vi "video.add.request.vi"(8 "error in":errorcluster, 9 "Series Tags":map{string, string}(c390), 10 "Video RID":string, 11 "DataScope Name":string="default") -> (0 "error out":errorcluster, 3 "Request":string)   [LabVIEW 2020, in "asset.lvclass"]
uses:
  d09293c4-a5fb-4d14-8e4d-efc786611564.vi
  dbf372a7-e192-454a-a0bf-8f356cd897b9.vi
  <vilib>/JDP Science/JSONtext/Variant to JSON Text.vi
  <vilib>/JDP Science/JSONtext/LVClass Serializer/JSONtext LVClass Serializer.lvclass
  nominal types/properties/properties.lvclass
  asset.lvclass
  asset.lvclass/asset.ctl
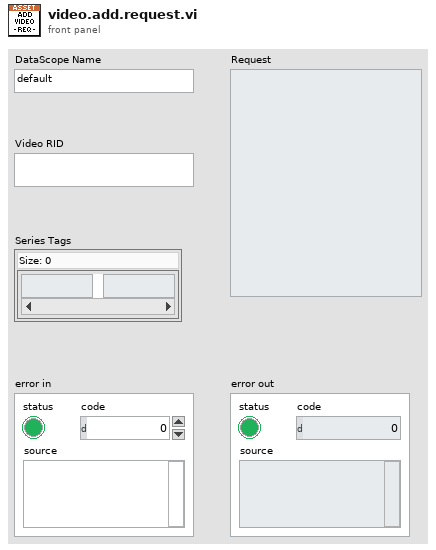
[diagram p1: front panel]
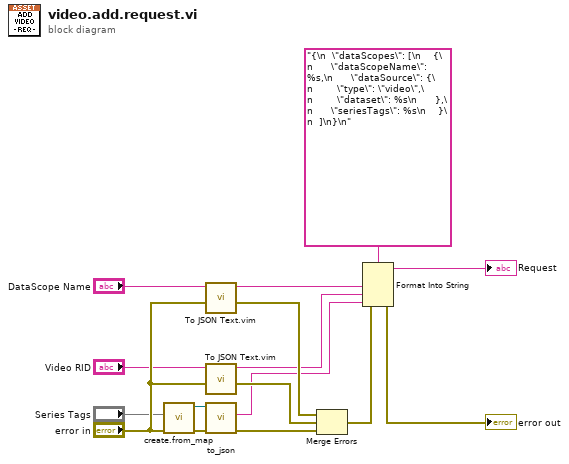
[diagram p0: block diagram]
diagram:
  n1 = call "create.from_map.vi"("error in"="error in", "properties"="Series Tags") -> ("error out"=w13:errorcluster, "properties out"=w14:refnum<class "properties.lvclass">)  [unwired: 8 in]
  n2 = call "To JSON Text.vim"("error in (no error)"="error in", "Anything"="DataScope Name") -> ("error out"=w16:errorcluster, "<JSON>"=w6:string)  [unwired: 8 in]
  n3 = call "To JSON Text.vim"("error in (no error)"="error in", "Anything"="Video RID") -> ("error out"=w15:errorcluster, "<JSON>"=w5:string)  [unwired: 8 in]
  n4 = call-dynamic "to_json.vi"("error in"=w13, "properties in"=w14) -> ("error out"=w8:errorcluster, "json"=w4:string)  [unwired: 6 in, 2 out]
  n5 = Merge Errors(w16, w15, w8) -> (w3:errorcluster)
  n6 = Format Into String(format string="{\n  \"dataScopes\": [\n    {\n      \"dataScopeName\": %s,\n      \"dataSource\": {\n        \"type\": \"video\",\n        \"dataset\": %s\n      },\n      \"seriesTags\": %s\n    }\n  ]\n}\n", error in=w3, w6, w5, w4) -> (resulting string=→"Request":string, error out=→"error out":errorcluster)  [unwired: 1 in]
